vi "CheckError.vi"(8 "State In":T1, 9 "Error In":errorcluster) -> (0 "State Out":T1, 1 "Error Out":errorcluster)   [LabVIEW 2020]
doc: "This VI check state machine state for error handler when error ocurres."
uses:
  Ctrls/StateMachineEnum.ctl
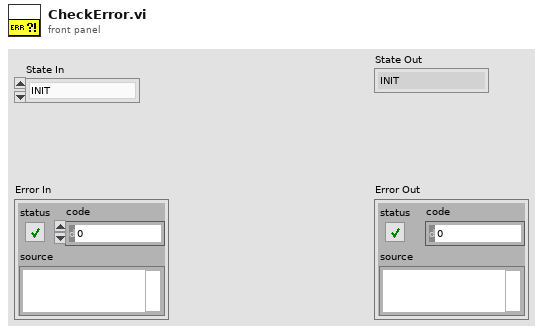
[diagram p1: front panel]
types:
  T1 = typedef "StateMachineEnum.ctl" = enum16{"INIT", "IDLE", "GET DATA", "ERROR HANDLER", "CLOSE"}
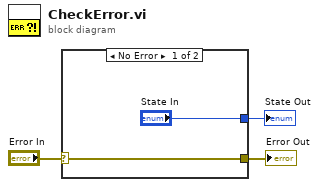
[diagram p0: block diagram]
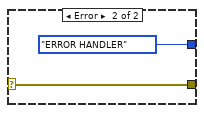
[diagram p2: hidden frame]
diagram:
  n1 = case shown="No Error" "Error In" {
    selector: "Error In" -> [w5 w6]
    tunnel: [w5 w6] -> w2
    tunnel: ["State In" StateMachineEnum."ERROR HANDLER" ("State In")] -> w1
    frame No Error {
    }
    frame Error {
    }
  }
  "Error Out" <- w2
  "State Out" <- w1
